vi "Fake Dust Head Control.vi"() -> ()   [LabVIEW 2009, in "Testing.lvlib"]
uses:
  Testing.lvlib
  interface/Dust Head.ctl
  interface/Interface.lvlib
panel:
  out "Iterations":i32
  in  "Rate (Hz)":dbl=1.0
  in  "stop":bool
  out "error out":errorcluster
  out "Out":T1
  in  "In":T1={"Lens"=12.5, "Needle/Housing"=7.0, "Pulse Frequency"=100.0, "Pulse Height"=2.1, "Pulse Width"=3.0}
  # "Fake Dust Head Control"
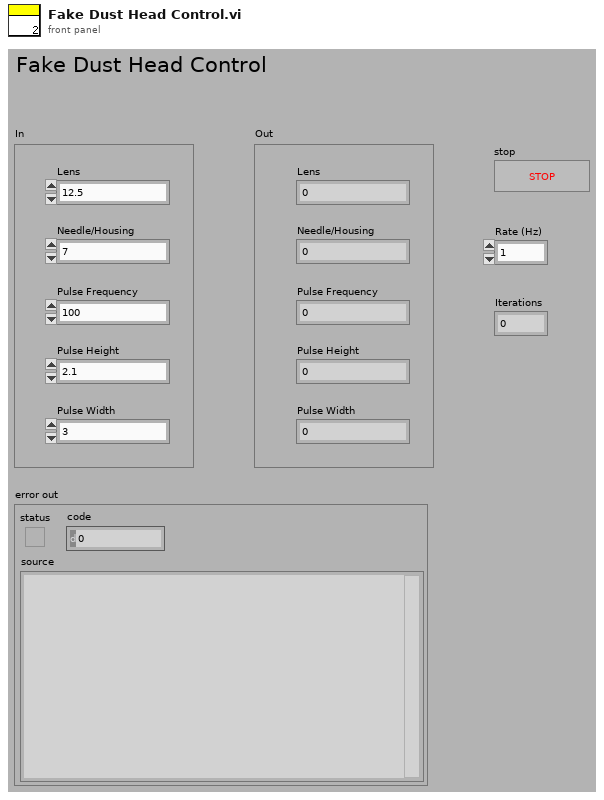
[diagram p1: front panel]
types:
  T1 = typedef "Interface.lvlib/Dust Head.ctl" = cluster{"Lens":dbl, "Needle/Housing":dbl, "Pulse Frequency":dbl, "Pulse Height":dbl, "Pulse Width":dbl}
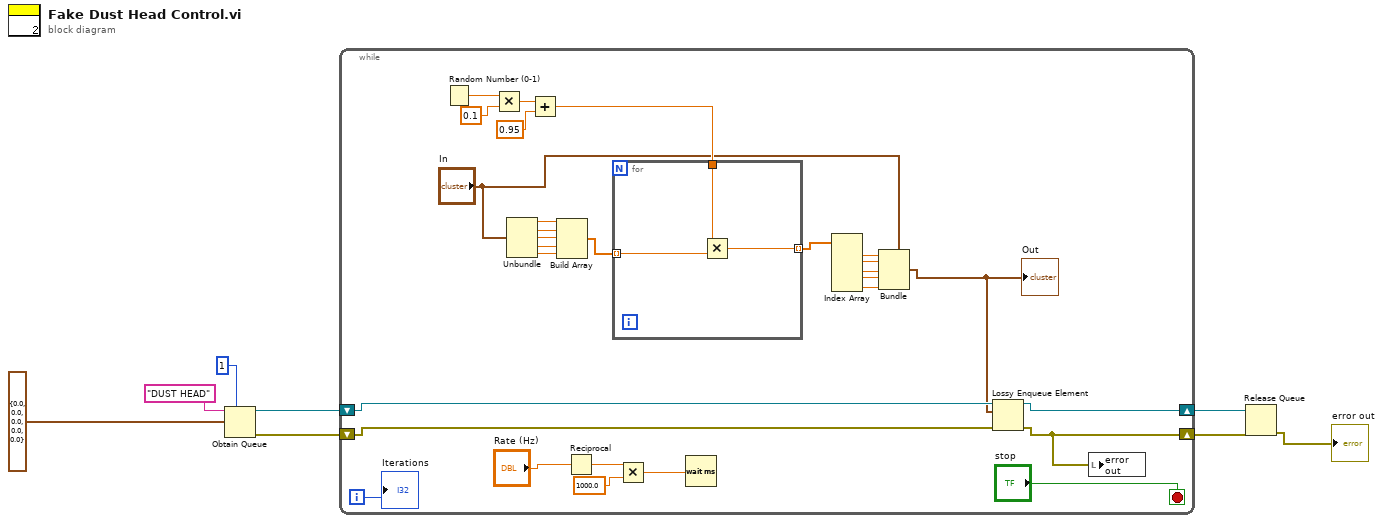
[diagram p0: block diagram]
diagram:
  n1 = Obtain Queue(max queue size (-1, unlimited)=1, name (unnamed)="DUST HEAD", element data type=T1 {"Lens"=0.0, "Needle/Housing"=0.0, "Pulse Frequency"=0.0, "Pulse Height"=0.0, "Pulse Width"=0.0} ("Cluster")) -> (queue out=w5:refnum<queue>, error out=w4:errorcluster)  [unwired: 2 in, 1 out]
  n2 = while {
    shift-right: [w15] -> w2
    shift-left: w4 -> [w18]
    shift-right: [w16] -> w3
    shift-left: w5 -> [w19]
    i -> [w13]
    stop <- "stop" stop-if-true
    n3 = Random Number (0-1)() -> (number: 0 to 1=w31:dbl)
    n4 = Multiply(x=w31, y=0.1) -> (x*y=w29:dbl)
    n5 = Unbundle("In") -> ("Lens"=w37:dbl, "Needle/Housing"=w36:dbl, "Pulse Frequency"=w35:dbl, "Pulse Height"=w34:dbl, "Pulse Width"=w33:dbl)
    n6 = Add(x=w29, y=0.95) -> (x+y=w27:dbl)
    n7 = Build Array(w37, w36, w35, w34, w33) -> (w32:dbl[])
    n8 = Reciprocal(x="Rate (Hz)") -> (1/x=w11:dbl)
    n9 = for {
      tunnel: w32 -> [w39] mode=indexing
      tunnel: w27 -> [w40]
      tunnel: [w38] -> w25 mode=indexing
      n10 = Multiply(x=w40, y=w39) -> (x*y=w38:dbl)
    }
    n11 = Multiply(x=w11, y=1000.0) -> (x*y=w9:dbl)
    n12 = Wait (ms)(milliseconds to wait=w9) -> ()  [unwired: 1 out]
    n13 = Index Array(array=w25) -> (element #1=w24:dbl, element #2=w23:dbl, element #3=w22:dbl, element #4=w21:dbl, element #5=w20:dbl)  [unwired: 5 in]
    n14 = Bundle(cluster="In", "Lens"=w24, "Needle/Housing"=w23, "Pulse Frequency"=w22, "Pulse Height"=w21, "Pulse Width"=w20) -> (w17:T1)
    "Out" <- w17
    n15 = Lossy Enqueue Element(queue=w19, element=w17, error in (no error)=w18) -> (queue out=w16:refnum<queue>, error out=w15:errorcluster)  [unwired: 2 out]
    n16 = local write "error out"(w15) -> ()
    "Iterations" <- w13
  }
  n17 = Release Queue(queue=w3, error in (no error)=w2) -> (error out=→"error out":errorcluster)  [unwired: 1 in, 2 out]
